vi "SLB - Door Control.vi"(0 "GEA2 Reference In":refnum<k24>, 7 "Action":enum16{"Close", "Open"}(ring), 11 "Error In":errorcluster) -> (4 "GEA2 Reference Out":refnum<k24>, 6 "Pass/Fail?":bool, 8 "Report Text":string, 15 "Error Out":errorcluster)   [LabVIEW 2016]
doc: "Use this VI to lock or unlock the lid."
uses:
  Q:/Common/DLLs/GEA3/GeaCommunication.dll
  Common/DLLs/GEA3/GeaCommunication.dll
  Common/LabVIEW GEA2 Toolkit/LabVIEW_GEA2_Toolkit.lvlibp/type defs/Source_Destination.ctl
  Common/LabVIEW GEA2 Toolkit/LabVIEW_GEA2_Toolkit.lvlibp/type defs/ERD Read Data In.ctl
  Common/LabVIEW GEA2 Toolkit/LabVIEW_GEA2_Toolkit.lvlibp/type defs/Data Type.ctl
  Common/LabVIEW GEA2 Toolkit/LabVIEW_GEA2_Toolkit.lvlibp
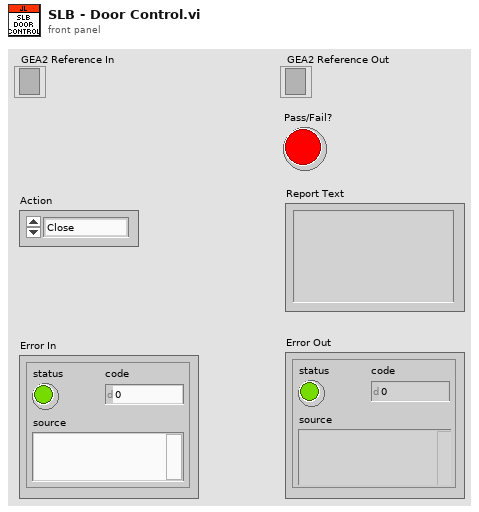
[diagram p1: front panel]
types:
  T1 = typedef "LabVIEW_GEA2_Toolkit.lvlibp/ERD Read Data In.ctl" = cluster{"ERD Number":u16, "Data Type":T2}
  T2 = typedef "LabVIEW_GEA2_Toolkit.lvlibp/Data Type.ctl" = enum16{"string", "boolean", "uint8_t", "uint16_t", "uint32_t", "uint64_t", "int8_t", "int16_t", "int32_t", "int64_t"}
  T3 = enum16{"EQ (==)", "NE (!=)", "GT (>)", "LT (<)", "GE (>=)", "LE (<=)", "GTLT(> <)", "GELE (>= <=)", "GELT (>= <)", "GTLE (> <=)", "LTGT (< >)", "LEGE (<= >=)", "LEGT (<= >)", "LTGE (< >=)", "No Comparison"}
  T4 = typedef "LabVIEW_GEA2_Toolkit.lvlibp/Source_Destination.ctl" = cluster{"Source":u8, "Destination":u8}
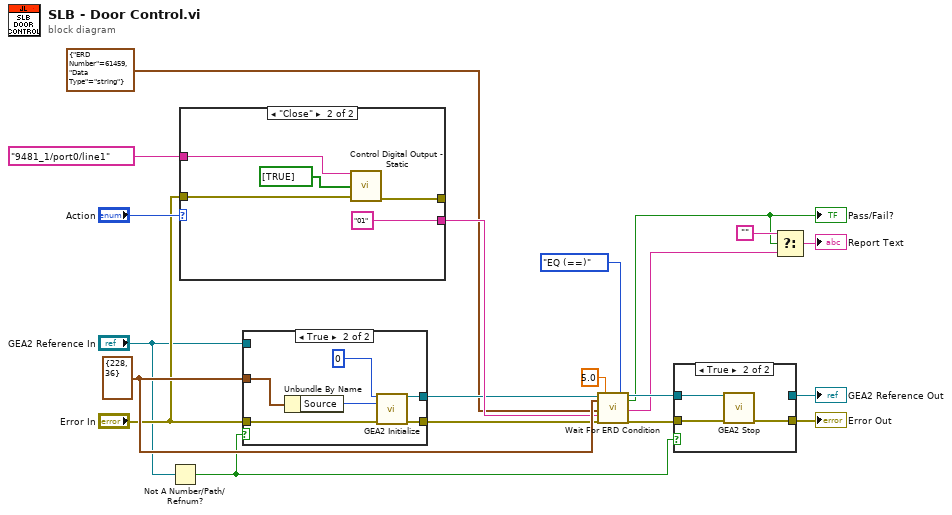
[diagram p0: block diagram]
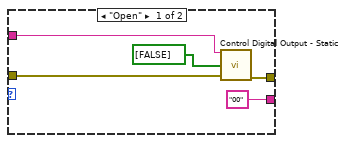
[diagram p2: hidden frame]
diagram:
  w18 = T4 {"Source"=228, "Destination"=36} ("GEA Inputs")
  n1 = Not A Number/Path/Refnum?(number/path/refnum="GEA2 Reference In") -> (NaN/Path/Refnum?=w2:bool)
  n2 = case shown="\"Close\"" "Action" {
    tunnel: ["00" ("y") "01" ("y")] -> w12
    tunnel: "Error In" -> [w24 w29]
    tunnel: [w23 w28] -> _
    tunnel: tag "9481_1/port0/line1" ("Line(s)") -> [w21 w26]
    frame "Open" {
      n3 = call "Control Digital Output - Static.vi"("Line(s)"=w21, "Output Array"=bool[] [FALSE], "Error In"=w24) -> ("Error Out"=w23:errorcluster)  [unwired: 12 in]
    }
    frame "Close" {
      n4 = call "Control Digital Output - Static.vi"("Line(s)"=w26, "Output Array"=bool[] [TRUE], "Error In"=w29) -> ("Error Out"=w28:errorcluster)  [unwired: 12 in]
    }
  }
  n5 = case shown="True" w2 {
    tunnel: "Error In" -> [w31 w38]
    tunnel: [w31 w37] -> w8
    tunnel: "GEA2 Reference In" -> [w32 _]
    tunnel: [w32 w36] -> w7
    tunnel: w18 -> [_ w34]
    frame False {
    }
    frame True {
      n6 = Unbundle By Name(w34) -> ("Source"=w35:u8)
      n7 = call "GEA2 Initialize.vi"("Board Index"=0, "Source Address"=w35, "error in"=w38) -> ("GEA2 Reference Out"=w36:refnum<k24>, "error out"=w37:errorcluster)  [unwired: 10 in, 1 out]
    }
  }
  n8 = call "Wait For ERD Condition.vi"("GEA2 Reference In"=w7, "GEA Inputs"=w18, "ERD Read Data"=T1 {"ERD Number"=61459, "Data Type"=enum."string"} ("ERD Read Data In"), "Expected Low"=w12, "Error In"=w8, "Timeout (s)"=5.0, "Comparison"=T3."EQ (==)") -> ("GEA2 Reference Out"=w17:refnum<k24>, "Pass/Fail?"=w11:bool, "Report Text"=w10:string, "Error Out"=w16:errorcluster)  [unwired: 8 in, 1 out]
  "Pass/Fail?" <- w11
  n9 = case shown="True" w2 {
    tunnel: w16 -> [w40 w43]
    tunnel: [w40 w42] -> w20
    tunnel: [w39 _] -> w19
    tunnel: w17 -> [w39 w41]
    frame False {
    }
    frame True {
      n10 = call "GEA2 Stop.vi"("GEA2 Reference In"=w41, "Error In"=w43) -> ("Error Out"=w42:errorcluster)  [unwired: 13 in]
    }
  }
  "Error Out" <- w20
  "GEA2 Reference Out" <- w19
  n11 = Select(t="", s=w11, f=w10) -> (s? t:f=→"Report Text":string)
